vi "Stop.vi"(8 "error in":errorcluster, 11 "Variant":variant) -> (0 "error out":errorcluster)   [LabVIEW 2020]
uses:
  Queue/Controls/Queue.ctl
  Queue/Controls/Queue_Mode.ctl
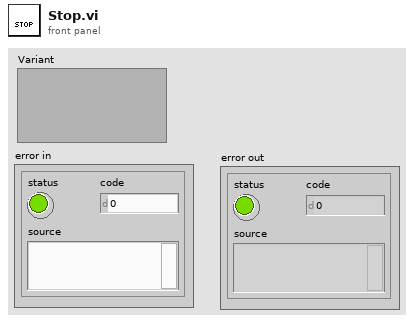
[diagram p1: front panel]
types:
  T1 = typedef "Queue.ctl" = cluster{"Mode":T2, "Data":variant}
  T2 = typedef "Queue_Mode.ctl" = enum16{"Start", "Stop"}
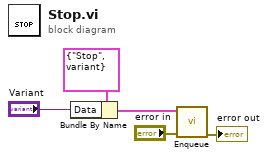
[diagram p0: block diagram]
diagram:
  n1 = Bundle By Name(cluster=T1 {"Mode"=enum."Stop", "Data"=variant} ("element"), "Data"="Variant") -> (w4:T1)
  n2 = call "Enqueue.vi"("error in"="error in", "element"=w4) -> ("error out"=→"error out":errorcluster)  [unwired: 9 in]
